vi "init.vi"(8 "error in":errorcluster, 11 "Controller S/N":string="0") -> (0 "error out":errorcluster)   [LabVIEW 2017]
panel:
  out "Conn. Axis":string[](array[string])
  out "Identification":string
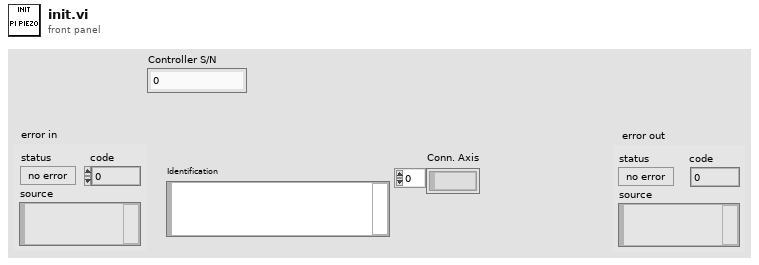
[diagram p1: front panel]
types:
  T1 = cluster{"RS232 settings":cluster{"Portnumber":i32, "Baudrate":u16}, "USB settings":cluster{"S/N":string, "USB Search?":bool}, "TCP/IP settings":cluster{"Host address/name":string, "Port":i32, "Board":i32, "TCP/IP Search?":bool}}
  T2 = cluster{"Check FRF?":bool, "Referencing mode":enum16{"FRF (-> FNL)", "FRF", "FNL", "FPL", "RON OFF"}[]}
  T3 = cluster{"Force?":bool, "Dialog?":bool, "Stages":string[]}
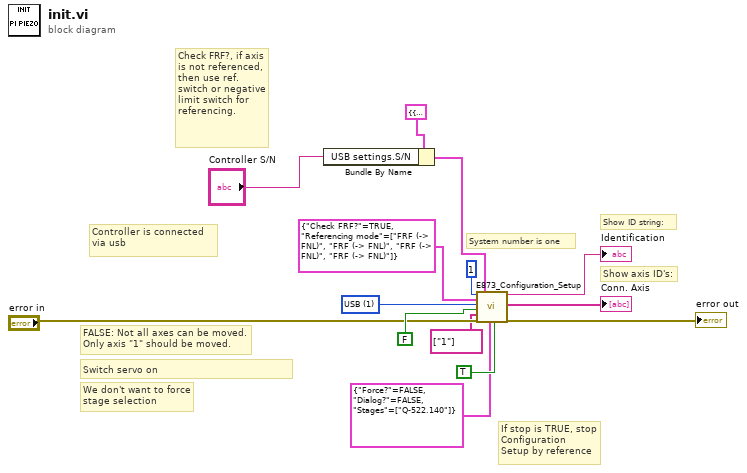
[diagram p0: block diagram]
diagram:
  w6 = u16 1 items=["RS232", "USB", "TCP/IP"] ("Interface")
  # "Check FRF?, if axis is not referenced, then use ref. switch or negative limit switch for referencing."
  # "We don't want to force\nstage selection"
  # "Controller is connected via usb"
  # "If stop is TRUE, stop \nConfiguration\nSetup by reference"
  # "Show axis ID's:"
  # "Show ID string:"
  # "Switch servo on"
  # "FALSE: Not all axes can be moved.\nOnly axis \"1\" should be moved."
  # "System number is one"
  n1 = Bundle By Name(cluster=T1 {"RS232 settings"={"Portnumber"=0, "Baudrate"=5}, "USB settings"={"S/N"="0", "USB Search?"=FALSE}, "TCP/IP settings"={"Host address/name"="localhost", "Port"=50000, "Board"=0, "TCP/IP Search?"=FALSE}} ("Interface settings"), "USB settings.S/N"="Controller S/N") -> (w2:T1)
  n2 = call "E873_Configuration_Setup.vi"("System no."=1, "Referencing"=T2 {"Check FRF?"=TRUE, "Referencing mode"=[enum."FRF (-> FNL)", enum."FRF (-> FNL)", enum."FRF (-> FNL)", enum."FRF (-> FNL)"]}, "Interface"=w6, "All axes?"=FALSE, "Axes to move"=string[] ["1"], "error in"="error in", "Interface settings"=w2, "Stage selection"=T3 {"Force?"=FALSE, "Dialog?"=FALSE, "Stages"=["Q-522.140"]}, "Switch servo on?"=TRUE ("Use dialog to define\nconnected stages?")) -> ("Identification"=→"Identification":string, "Conn. \nAxes"=→"Conn. Axis":string[], "error out"=→"error out":errorcluster)  [unwired: 3 in, 5 out]
